vi "Get Alarm State.vi"(11 "Pump_1AI_1DO_2DI in":refnum<class "Valve_2DO_2DI.lvclass">) -> (2 "Alarm State":bool)   [LabVIEW 2019, in "Valve_2DO_2DI.lvclass"]
uses:
  Valve_2DO_2DI.lvclass
  Valve_2DO_2DI.lvclass/Valve_2DO_2DI.ctl
  DA_class/DA.lvclass/DA.ctl
  DA_class/DA.lvclass
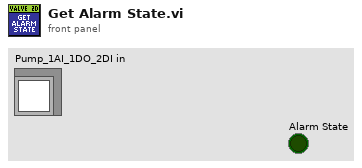
[diagram p1: front panel]
types:
  T1 = typedef "bool_data.ctl" = cluster{"CURR":bool, "RAW_PREV":bool, "millisecond timer value":u32}
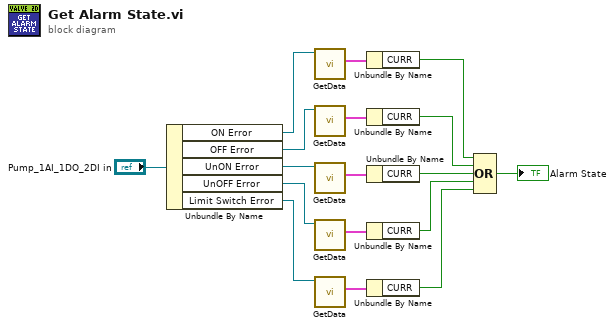
[diagram p0: block diagram]
diagram:
  n1 = Unbundle By Name("Pump_1AI_1DO_2DI in") -> ("ON Error"=w16:refnum<class "DA.lvclass">, "OFF Error"=w11:refnum<class "DA.lvclass">, "UnON Error"=w10:refnum<class "DA.lvclass">, "UnOFF Error"=w9:refnum<class "DA.lvclass">, "Limit Switch Error"=w2:refnum<class "DA.lvclass">)
  n2 = call "GetData.vi"("Sig_DA in"=w16) -> ("data"=w15:T1)  [unwired: 10 in]
  n3 = call "GetData.vi"("Sig_DA in"=w11) -> ("data"=w14:T1)  [unwired: 10 in]
  n4 = call "GetData.vi"("Sig_DA in"=w10) -> ("data"=w13:T1)  [unwired: 10 in]
  n5 = call "GetData.vi"("Sig_DA in"=w9) -> ("data"=w12:T1)  [unwired: 10 in]
  n6 = call "GetData.vi"("Sig_DA in"=w2) -> ("data"=w3:T1)  [unwired: 10 in]
  n7 = Unbundle By Name(w15) -> ("CURR"=w8:bool)
  n8 = Unbundle By Name(w14) -> ("CURR"=w7:bool)
  n9 = Unbundle By Name(w13) -> ("CURR"=w6:bool)
  n10 = Unbundle By Name(w12) -> ("CURR"=w5:bool)
  n11 = Unbundle By Name(w3) -> ("CURR"=w1:bool)
  n12 = Compound Arithmetic op=OR(w8, w7, w6, w5, w1) -> (→"Alarm State":bool)
